vi "Micro-PL v10.1.0.vi"() -> ()   [LabVIEW 2010]
uses:
  drivers/Oxford ITC/ITCAPPS.LLB/ITCSetup.ctl
  drivers/Oxford ITC/ITCSUBS.LLB/ITCIO.ctl
  drivers/Oxford ITC/BUSGEN.LLB/OxfordAddress.ctl
  drivers/Oxford ITC/ITCSUBS.LLB/ITCVersion.ctl
  subvi/ESA-C/TypeDefs/ESA-C Live Controls.ctl
  subvi/ESA-C/TypeDefs/ESA-C Current Values.ctl
  subvi/ESA-C/TypeDefs/ESA-C Connection Settings.ctl
  subvi/ESA-C/TypeDefs/ESA-C Set Positions.ctl
  subvi/ITC503/TypeDefs/ITC503 Settings.ctl
  subvi/ITC503/TypeDefs/ITC503 Current Values.ctl
  subvi/iHR550/TypeDefs/iHR Current Values.ctl
  subvi/iHR550/TypeDefs/iHR Settings.ctl
  subvi/Mapping/TypeDefs/Mapping Spectra Params.ctl
  <vilib>/Utility/miscctls.llb/LVPointTypeDef.ctl
  drivers/Horiba Spectrum One 3000V/Lib/CCD_command.llb/Comm Params.ctl
panel:
  out "Int. Time Temp":dbl
  out "Wavelengths (nm)":dbl[](array[numeric])
  out "Measurement Running":bool
  out "ITC503s Running":bool
  out "Drive Running":bool
  out "CCD3500V Running":bool
  out "iHR550 Running":bool
  in  "Exit":bool
  out "iHR550 Status":bool
  out "Drive Status":bool
  out "CCD3500V Status":bool
  out "ITC503 Status":bool
  in  "CCD3500V Connection":T1={"Comm Interface"=1, "BUS"=0, "Address"=5, "Com Port"=0}
  out "Video Running":bool
  out "iHR550 RefNum":refnum<k7> caption="Mono RefNum out"
  out "ITC Setup":T2={"Description"="", "IO Info"={"Address"={"Com Port"=1, "ISOBUS Address"=1, "GPIB Address"=24, "Communication"=enum."ISOBUS"}, "Version"=enum."ITC503", "Ch 1 dec places"=1, "Ch 2 dec places"=1, "Ch 3 dec places"=1, "Ch1 Name"="", "Ch2 Name"="", "Ch3 Name"=""}}
  in  "Register":T6(tab)
  in  "iHR550 Force Init":bool=TRUE
  in  "iHR550 Connect":bool
  in  "iHR550 ID":string(combo)="iHR550" caption="Monochromator ID"
  out "ITC503 Current Values":T7 {"ITC503 Gradient" format="%.2f"; "ITC503 Setpoint" min=-273.0 max=300000.0 step=0.0001 format="%.1f"; "ITC503 I" format="%_1f"; "ITC503 P" format="%_1f"; "ITC503 Temperature" min=0.0 max=1645.0 step=1e-05 format="%.2f"; "ITC503 Heater" min=0.0 max=100.0 step=0.01 scale=0.0..100.0}
  in  "ITC503 Settings":T8={"ITC503 Set Setpoint"=0.0, "ITC503 Set Auto Heater"=TRUE, "ITC503 Set Auto PID"=TRUE, "P"=0.0, "I"=0.0, "D"=0.0} {"D" min=0.0 max=100.0 step=0.1 format="%.1f"; "I" min=0.0 max=100.0 step=0.1 format="%.1f"; "P" min=0.0 max=100.0 step=0.1 format="%.1f"; "ITC503 Set Setpoint" min=-273.0 max=300000.0 step=0.1 format="%.1f"}
  in  "ITC503 Configure":bool
  in  "ITC503 Connect":bool
  in  "ITC503 Selector":u16(ring) caption="Select Device" items=["ITC503s"]
  out "Drive Current Values":T9 {"Position"."Drive Z Position" min=-273.0 max=300000.0 step=0.0001 format="%.1f"; "Position"."Drive Y Position" min=-273.0 max=300000.0 step=0.0001 format="%.1f"; "Position"."Drive X Position" min=-273.0 max=300000.0 step=0.0001 format="%.1f"; "Voltages"."Drive Z Voltage" min=-273.0 max=300000.0 step=0.0001 format="%.1f"; "Voltages"."Drive Y Voltage" min=-273.0 max=300000.0 step=0.0001 format="%.1f"; "Voltages"."Drive X Voltage" min=-273.0 max=300000.0 step=0.0001 format="%.1f"}
  in  "Drive Connection":T10={"Objective GPIB-Port"=4, "Stage GPIB-Port"=4, "Drive Selector"=0, "Drive Velocity (V/s)"=5.0} {"Drive Velocity (V/s)" min=10.0 max=160.0 step=0.1 format="%.1f"; "Drive Selector" items=["Obj.", "Stage"]; "Stage GPIB-Port" min=1 max=20 step=1 format="%#.0f"; "Objective GPIB-Port" min=1 max=20 step=1 format="%#.0f"}
  in  "Drive Connect":bool
  out "CCD3500 Temperature":dbl caption="Temp. (°C)" min=10.0 max=160.0 step=0.1 format="%.1f"
  in  "CCD3500V GPIB-Port":i32=5 caption="GPIB-Port" min=1 max=20 step=1 format="%#.0f"
  in  "CCD3500V Connect":bool
  in  "CCD3000 Current Rep.":string="0/0"
  in  "Spectrum Load":bool
  in  "Spectrum Save":bool
  out "Spectrum":cluster{dbl[], dbl[]}[](graph)
  in  "Video Show":bool
  in  "Drive GoTo":bool caption="Objective Move Abs."
  in  "Drive New Positions":T11 {"Drive X Set" min=10.0 max=160.0 step=0.1 format="%.1f"; "Drive Z Set" min=10.0 max=160.0 step=0.1 format="%.1f"; "Drive Y Set" min=10.0 max=160.0 step=0.1 format="%.1f"}
  in  "Spectrum Autosave":bool=TRUE caption="iHR550 Force Init"
  in  "CCD3500 Preview":bool
  in  "CCD3500 Acquire":bool
  in  "Spectra Settings":T12={"Integration Time"=1.0, "Repetitions"=1, "Mapping Spectra"=TRUE} caption="Mapping Spectra Settings" {"Repetitions" min=1 max=100 step=1; "Integration Time" min=0.1 max=6000.0 step=0.1 format="%.1f"}
  in  "Mapping Start":bool
  in  "iHR550 Configure":bool
  in  "iHR Settings":T13={"iHR550 Set Exit Mirror"=2, "iHR550 Set Side Exit"=0.0, "iHR550 Set Front Entrance"=0.0, "iHR550 Set Wavelength"=897.9988, "iHR550 Set Grating"=0, "iHR550 Set Grating Switch"=FALSE, "iHR550 Set Wavelength Switch"=FALSE, "iHR550 Set Mirror Switch"=FALSE, "iHR550 Set Slits Switch"=FALSE} {"iHR550 Set Grating" items=["1800"=1, "600"=2, "150"=3]; "iHR550 Set Wavelength" min=0.0 max=1500.0 step=1.0; "iHR550 Set Side Exit" min=0.0 max=2000.0 step=1.0; "iHR550 Set Exit Mirror" items=["Front"=2, "Side"=3]}
  out "iHR Current Values":T14={"iHR 550 Front Entrance"=0.0, "iHR550 Side Exit"=0.0, "iHR550 Wavelength"=897.9988, "iHR550 Exit Mirror"=2, "iHR550 Grating"="1", "Grating Index"=1} {"iHR550 Exit Mirror" items=["EntranceMirror", "ExitMirror", "Front", "Side"]}
  out "Drive Live Current Values":T9 {"Position"."Drive Z Position" min=-273.0 max=300000.0 step=0.0001 format="%.1f"; "Position"."Drive Y Position" min=-273.0 max=300000.0 step=0.0001 format="%.1f"; "Position"."Drive X Position" min=-273.0 max=300000.0 step=0.0001 format="%.1f"; "Voltages"."Drive Z Voltage" min=-273.0 max=300000.0 step=0.0001 format="%.1f"; "Voltages"."Drive Y Voltage" min=-273.0 max=300000.0 step=0.0001 format="%.1f"; "Voltages"."Drive X Voltage" min=-273.0 max=300000.0 step=0.0001 format="%.1f"}
  in  "Drive Live Controls":T15={"Snapshot"=FALSE, "Move Step"=1.0, "Move Home"=FALSE, "Move Down"=FALSE, "Move Up"=FALSE, "Move Left"=FALSE, "Move Right"=FALSE, "Move Out"=FALSE, "Move In"=FALSE} {"Move Step" min=0.0 max=30.0 step=0.1 format="%.1f"}
  # "Correlation Setup"
  # "Active"
  # "Active"
  # "ITC"
  # "iHR"
  # "Drive"
  # "CCD"
  # "Status"
  # "CCD"
  # "ITC"
  # "iHR"
  # "Drive"
  # "Monochromator"
  # "Cryostat"
  # "Drives"
  # "CCD-Camera"
  # "Drive Control"
  # "Spectrum"
  # "CCD"
  # "Mapping"
  # "Launch the Spectral Mapping VI and Raman Tool Set 2.0 in a new window."
  # "Monochromator"
  # "XY"
  # "Z"
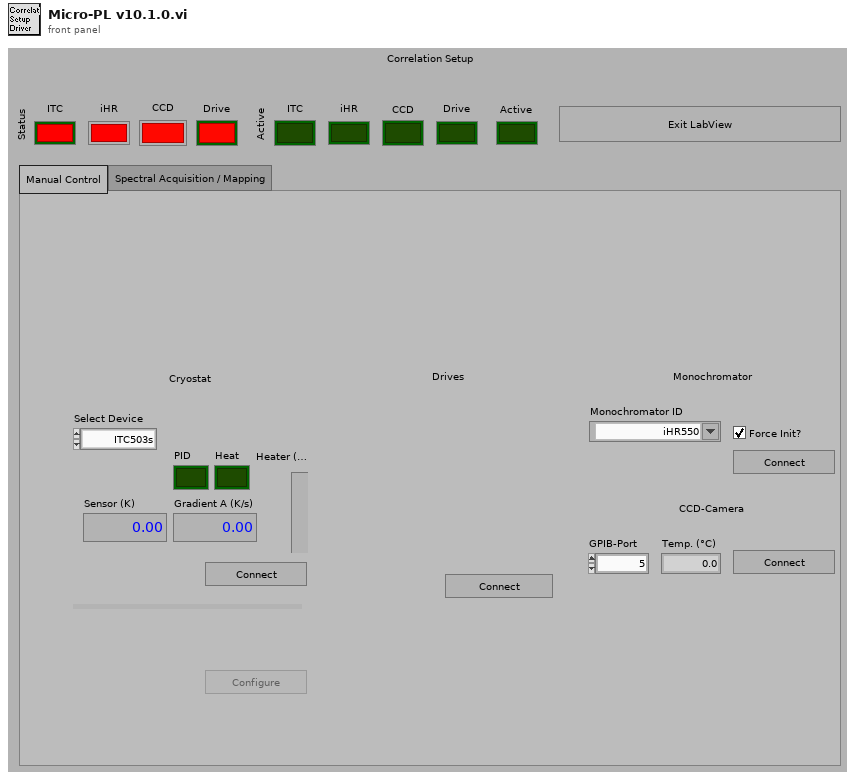
[diagram p1: front panel]
types:
  T1 = cluster{"Comm Interface":u16, "BUS":i16, "Address":i16, "Com Port":i32}
  T2 = typedef "ITCSetup.ctl" = cluster{"Description":string, "IO Info":T3}
  T3 = typedef "ITCIO.ctl" = cluster{"Address":T4, "Version":T5, "Ch 1 dec places":i16, "Ch 2 dec places":i16, "Ch 3 dec places":i16, "Ch1 Name":string, "Ch2 Name":string, "Ch3 Name":string}
  T4 = typedef "OxfordAddress.ctl" = cluster{"Com Port":i32, "ISOBUS Address":i32, "GPIB Address":i16, "Communication":enum16{"RS232", "ISOBUS", "GPIB", "Gateway"}}
  T5 = typedef "ITCVersion.ctl" = enum16{"ITC502", "ITC503", "ITC601"}
  T6 = enum32{"Manual Control", "Spectral Acquisition / Mapping"}
  T7 = typedef "ITC503 Current Values.ctl" = cluster{"ITC503 Heater":dbl, "ITC503 Temperature":dbl, "ITC503 P":dbl, "ITC503 I":dbl, "ITC503 D":dbl, "ITC503 Setpoint":dbl, "ITC503 Gradient":dbl, "ITC503 Heater Auto":bool, "ITC503 PID Auto":bool}
  T8 = typedef "ITC503 Settings.ctl" = cluster{"ITC503 Set Setpoint":dbl, "ITC503 Set Auto Heater":bool, "ITC503 Set Auto PID":bool, "P":dbl, "I":dbl, "D":dbl}
  T9 = typedef "ESA-C Current Values.ctl" = cluster{"Voltages":cluster{"Drive X Voltage":dbl, "Drive Y Voltage":dbl, "Drive Z Voltage":dbl}, "Position":cluster{"Drive X Position":dbl, "Drive Y Position":dbl, "Drive Z Position":dbl}}
  T10 = typedef "ESA-C Connection Settings.ctl" = cluster{"Objective GPIB-Port":i32, "Stage GPIB-Port":i32, "Drive Selector":u16, "Drive Velocity (V/s)":dbl}
  T11 = typedef "ESA-C Set Positions.ctl" = cluster{"Drive X Set":dbl, "Drive Y Set":dbl, "Drive Z Set":dbl}
  T12 = typedef "Mapping Spectra Params.ctl" = cluster{"Integration Time":dbl, "Repetitions":u16, "Mapping Spectra":bool}
  T13 = typedef "iHR Settings.ctl" = cluster{"iHR550 Set Exit Mirror":u16, "iHR550 Set Side Exit":dbl, "iHR550 Set Front Entrance":dbl, "iHR550 Set Wavelength":dbl, "iHR550 Set Grating":u16, "iHR550 Set Grating Switch":bool, "iHR550 Set Wavelength Switch":bool, "iHR550 Set Mirror Switch":bool, "iHR550 Set Slits Switch":bool}
  T14 = typedef "iHR Current Values.ctl" = cluster{"iHR 550 Front Entrance":dbl, "iHR550 Side Exit":dbl, "iHR550 Wavelength":dbl, "iHR550 Exit Mirror":i32, "iHR550 Grating":string, "Grating Index":i32}
  T15 = typedef "ESA-C Live Controls.ctl" = cluster{"Snapshot":bool, "Move Step":dbl, "Move Home":bool, "Move Down":bool, "Move Up":bool, "Move Left":bool, "Move Right":bool, "Move Out":bool, "Move In":bool}
  T16 = typedef "LVPointTypeDef.ctl" = cluster{"Horizontal":i16, "Vertical":i16}
  T17 = enum16{"CCD Temperature Z345", "CCD Temperature Z308", "CCD Gain"}
  T18 = enum8{"Enabled", "Disabled", "Disabled and Grayed Out"}
  T19 = typedef "Comm Params.ctl" = cluster{"Comm Interface":u16, "BUS":i16, "Address":i16, "Com Port":i32}
  T20 = cluster{"CCD3000 Connection":T19, "Drive Connection Settings":T10, "ITC503 Current Values":T7, "Wavelengths (nm)":dbl[], "Drive Current Values":T9, "iHR Current Values":T14, "Spectra Settings":T12, "CCD3500 Temperature":dbl, "Simulate Drive 2":bool, "Simulate Spectra 2":bool}
  T21 = cluster{"Intensities":dbl[], "Wavelengths":dbl[]}[]
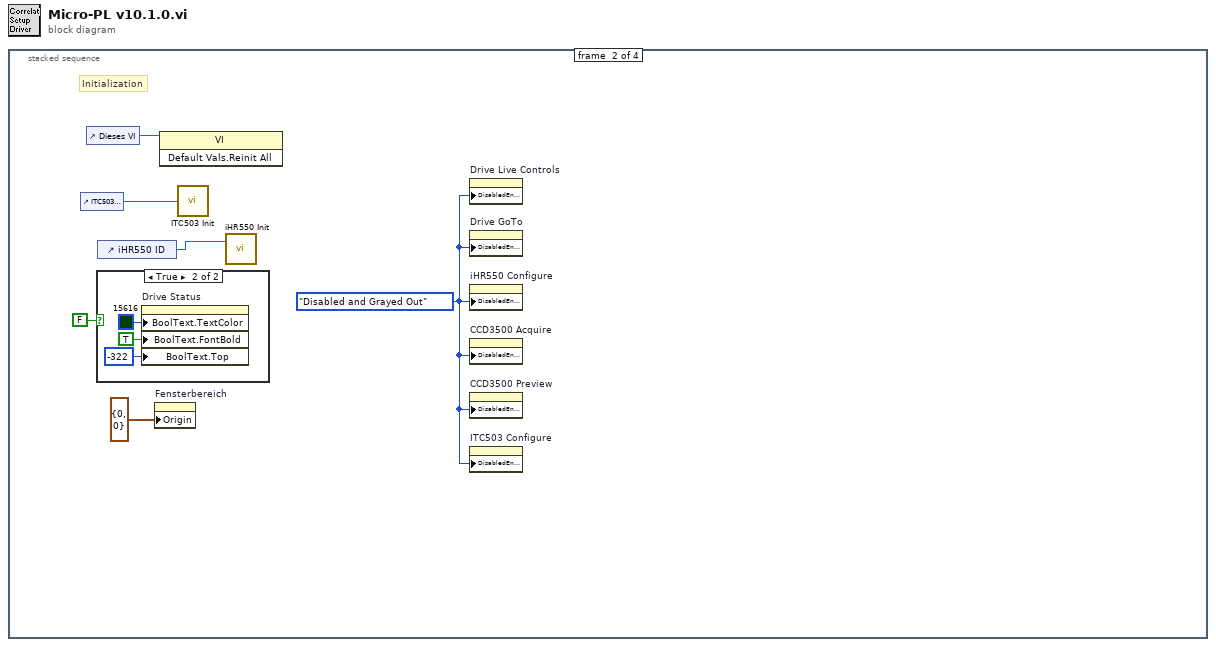
[diagram p0: block diagram]
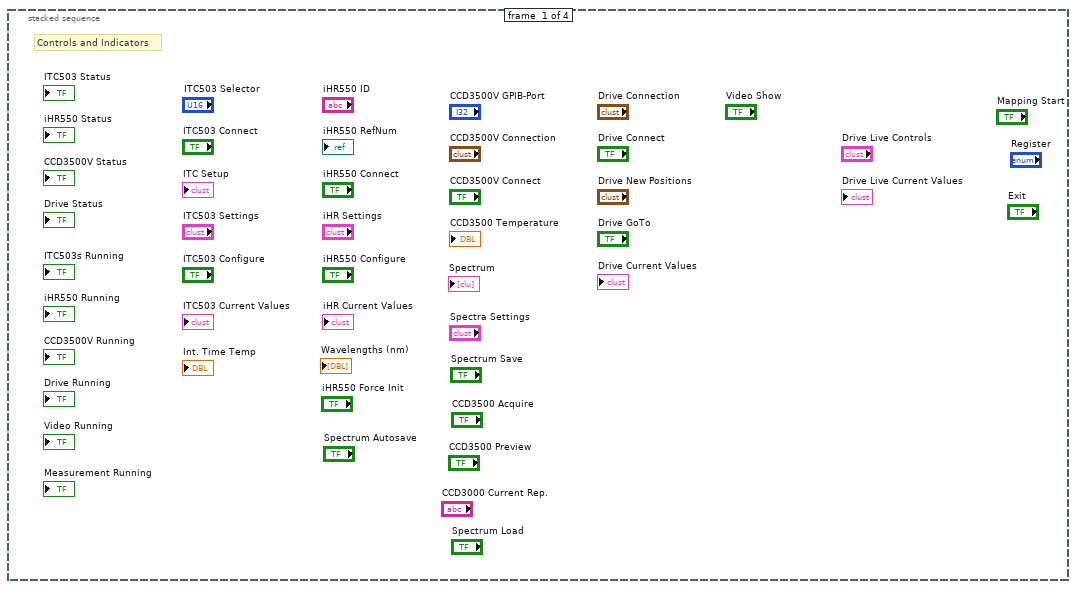
[diagram p2: hidden frame]
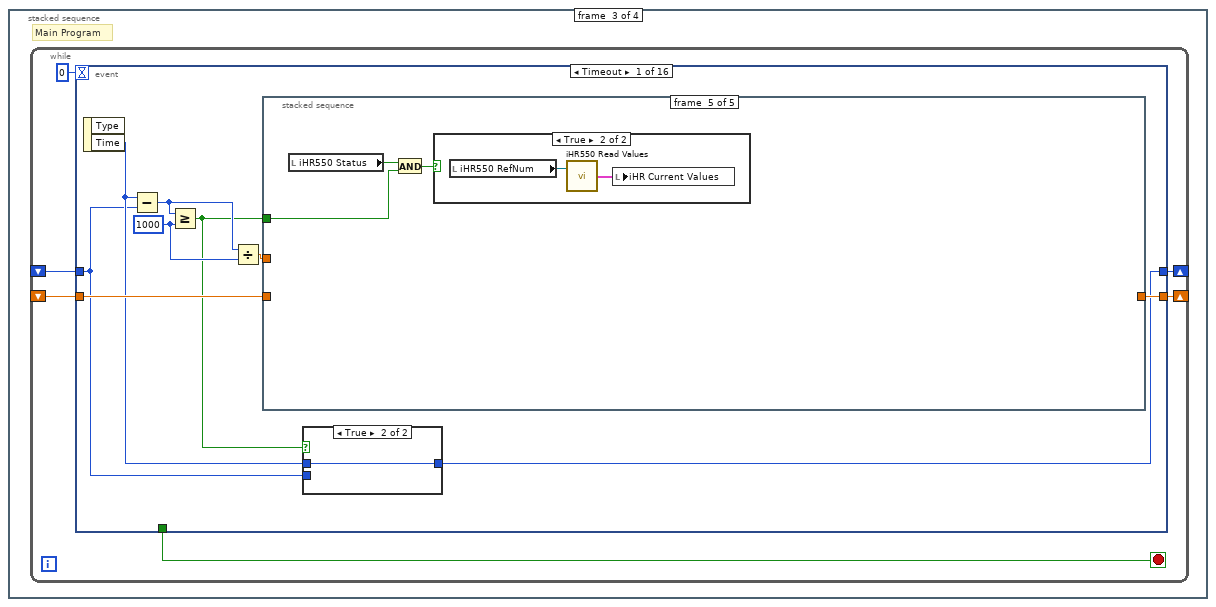
[diagram p4: hidden frame]
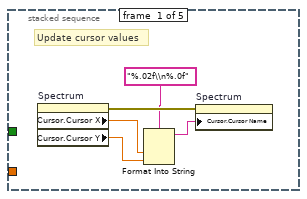
[diagram p6: hidden frame]
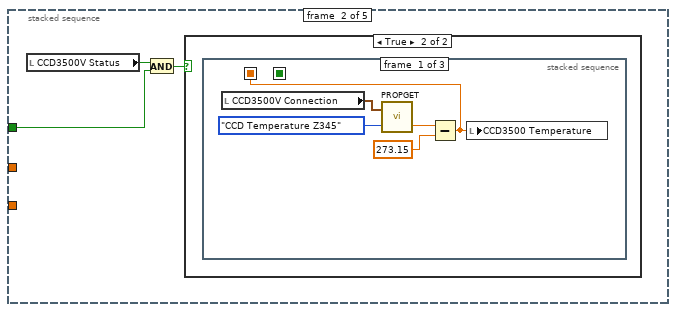
[diagram p7: hidden frame]
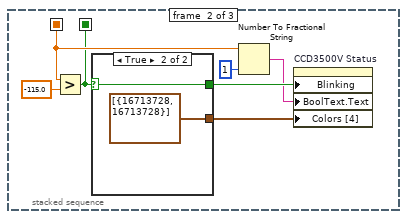
[diagram p9: hidden frame]
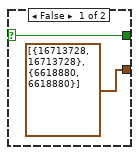
[diagram p10: hidden frame]
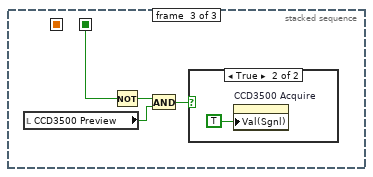
[diagram p11: hidden frame]
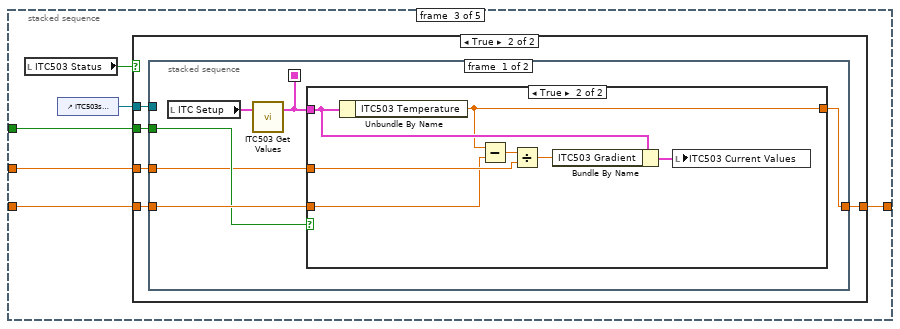
[diagram p13: hidden frame]
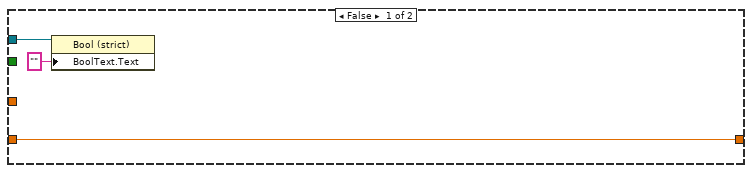
[diagram p14: hidden frame]
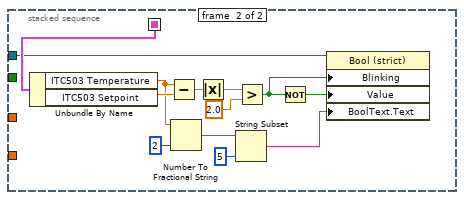
[diagram p16: hidden frame]
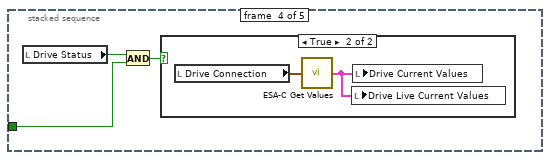
[diagram p17: hidden frame]
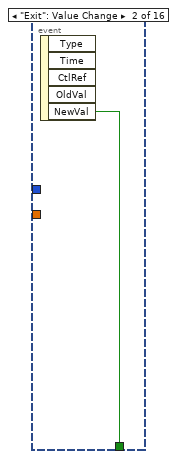
[diagram p20: hidden frame]
diagram:
  n1 = stacked-sequence {
    frame #0 {
      # "Controls and Indicators"
    }
    frame #1 {
      w1 = T18."Disabled and Grayed Out" ("Deaktiviert")
      # "Initialization"
      n2 = control-ref of="ITC503 Selector"() -> (w6:refnum<vi>)
      n3 = control-ref of="Dieses VI"() -> (w5:refnum<vi>)
      n4 = case shown="True" FALSE {
        frame False {
        }
        frame True {
          n5 = property on="Drive Status" class="Bool (strict)"("BoolText.TextColor"=u32 15616, "BoolText.FontBold"=TRUE ("Boolescher Text.Schriftart:Fett"), "BoolText.Top"=-322 ("Boolescher Text.Position:Oben")) -> ()  [unwired: 2 in, 2 out]
        }
      }
      n6 = control-ref of="iHR550 ID"() -> (w4:refnum<vi>)
      n7 = property on="Fensterbereich" class="Pane"("Origin"=T16 {"Horizontal"=0, "Vertical"=0}) -> ()  [unwired: 2 in, 2 out]
      n8 = invoke class="VI" method="Default Vals.Reinit All"(reference=w5) -> ()  [unwired: 2 in, 3 out]
      n9 = call "ITC503 Init.vi"("ITC Selector"=w6) -> ()  [unwired: 1 in]
      n10 = call "iHR550 Init.vi"("Mono ID"=w4) -> ()  [unwired: 2 in]
      n11 = property on="Drive Live Controls" class="Clust (strict)"("DisabledEnum"=w1) -> ()  [unwired: 2 in, 2 out]
      n12 = property on="Drive GoTo" class="Bool (strict)"("DisabledEnum"=w1) -> ()  [unwired: 2 in, 2 out]
      n13 = property on="iHR550 Configure" class="Bool (strict)"("DisabledEnum"=w1) -> ()  [unwired: 2 in, 2 out]
      n14 = property on="CCD3500 Acquire" class="Bool (strict)"("DisabledEnum"=w1) -> ()  [unwired: 2 in, 2 out]
      n15 = property on="CCD3500 Preview" class="Bool (strict)"("DisabledEnum"=w1) -> ()  [unwired: 2 in, 2 out]
      n16 = property on="ITC503 Configure" class="Bool (strict)"("DisabledEnum"=w1) -> ()  [unwired: 2 in, 2 out]
    }
    frame #2 {
      # "Main Program"
      n17 = while "Main-Program" {
        shift-right: [w13] -> _
        shift-left: _ -> [w12]
        shift-right: [w11] -> _
        shift-left: _ -> [w10]
        stop <- w15 stop-if-true
        n18 = event shown="[0] Timeout" {
          selector: _ -> [_ _ _ _ _ _ _ _ _ _ _ _ _ _ _ _]
          dyn-events: _ -> [_ _ _ _ _ _ _ _ _ _ _ _ _ _ _ _]
          timeout: 0 -> [_ _ _ _ _ _ _ _ _ _ _ _ _ _ _ _]
          tunnel: [_ w107 _ _ _ _ _ _ _ _ _ _ _ _ _ _] -> w15
          tunnel: w12 -> [w16 _ _ _ _ _ _ _ _ _ _ _ _ _ _ _]
          tunnel: [w17 _ _ _ _ _ _ _ _ _ _ _ _ _ _ _] -> w13
          tunnel: [w24 _ _ _ _ _ _ _ _ _ _ _ _ _ _ _] -> w11
          tunnel: w10 -> [w23 _ _ _ _ _ _ _ _ _ _ _ _ _ _ _]
          event Timeout {
            w21 = u32 1000 ("y")
            n19 = event-data() -> ("Time"=w18:u32)  [unwired: 1 in, 1 out]
            n20 = Subtract(x=w18, y=w16) -> (x-y=w22:u32)
            n21 = Greater Or Equal?(x=w22, y=w21) -> (x >= y?=w19:bool)
            n22 = Divide(x=w22, y=w21) -> (x/y=w20:dbl)
            n23 = stacked-sequence {
              tunnel: [_ _ w59 _ _] -> w24
              tunnel: w23 -> [_ _ w58 _ _]
              tunnel: w19 -> [_ w32 w57 w99 w103]
              tunnel: w20 -> [_ _ w56 _ _]
              frame #0 {
                # "Update cursor values"
                n24 = property on="Spectrum" class="XYGraph (strict)"() -> (error out=w31:errorcluster, "Cursor.Cursor X"=w30:dbl, "Cursor.Cursor Y"=w29:dbl)  [unwired: 2 in, 1 out]
                n25 = Format Into String(format string="%.02f\\n%.0f", w30, w29) -> (resulting string=w27:string)  [unwired: 2 in, 1 out]
                n26 = property on="Spectrum" class="XYGraph (strict)"(error in=w31, "Cursor.Cursor Name"=w27) -> ()  [unwired: 1 in, 2 out]
              }
              frame #1 {
                n27 = local read "CCD3500V Status"() -> (w34:bool)
                n28 = And(x=w34, y=w32) -> (x .and. y?=w33:bool)
                n29 = case shown="True" w33 {
                  frame False {
                  }
                  frame True {
                    n30 = stacked-sequence {
                      seq-local: [w35 _ _] -> [_ w44 _]
                      seq-local: [_ w40 _] -> [_ _ w54]
                      frame #0 {
                        n31 = local read "CCD3500V Connection"() -> (w39:T1)
                        n32 = call "PROPGET.VI"("CCD Prop ID"=T17."CCD Temperature Z345", "Comm Params"=w39) -> ("Output Param"=w37:dbl)  [unwired: 1 out]
                        n33 = Subtract(x=w37, y=273.15) -> (x-y=w35:dbl)
                        n34 = local write "CCD3500 Temperature"(w35) -> ()
                      }
                      frame #1 {
                        n35 = Greater?(x=w44, y=-115.0) -> (0:w40:bool)
                        n36 = case shown="True" w40 {
                          selector: w40 -> [w48 w50]
                          tunnel: [cluster{u32, u32}[] [{16713728, 16713728}, {6618880, 6618880}] ("Farben [4]") cluster{u32, u32}[] [{16713728, 16713728}] ("Farben [4]")] -> w41
                          tunnel: [w48 w50] -> w43
                          frame False {
                          }
                          frame True {
                          }
                        }
                        n37 = Number To Fractional String(number=w44, precision (6)=i16 1 ("Genauigkeit (6)")) -> (F-format string=w42:string)  [unwired: 2 in]
                        n38 = property on="CCD3500V Status" class="Bool (strict)"("Blinking"=w43, "BoolText.Text"=w42, "Colors [4]"=w41) -> ()  [unwired: 2 in, 2 out]
                      }
                      frame #2 {
                        n39 = local read "CCD3500 Preview"() -> (w52:bool)
                        n40 = Not(x=w54) -> (.not. x?=w53:bool)
                        n41 = And(x=w53, y=w52) -> (x .and. y?=w51:bool)
                        n42 = case shown="True" w51 {
                          frame False {
                          }
                          frame True {
                            n43 = property on="CCD3500 Acquire" class="Bool (strict)"("Val(Sgnl)"=TRUE ("Wert (signalisierend)")) -> ()  [unwired: 2 in, 2 out]
                          }
                        }
                      }
                    }
                  }
                }
              }
              frame #2 {
                n44 = local read "ITC503 Status"() -> (w61:bool)
                n45 = control-ref of="ITC503s Running"() -> (w60:refnum<vi>)
                n46 = case shown="True" w61 {
                  tunnel: w60 -> [w64 w69]
                  tunnel: [w62 w68] -> w59
                  tunnel: w58 -> [w62 w67]
                  tunnel: w57 -> [_ w66]
                  tunnel: w56 -> [_ w65]
                  frame False {
                    n47 = property class="Bool (strict)"(reference=w64, "BoolText.Text"="" ("Boolescher Text.Text")) -> ()  [unwired: 1 in, 2 out]
                  }
                  frame True {
                    n48 = stacked-sequence {
                      seq-local: [w74 _] -> [_ w92]
                      tunnel: w69 -> [_ w89]
                      tunnel: [w73 _] -> w68
                      tunnel: w67 -> [w72 _]
                      tunnel: w66 -> [w71 _]
                      tunnel: w65 -> [w70 _]
                      frame #0 {
                        n49 = local read "ITC Setup"() -> (w75:T2)
                        n50 = call "ITC503 Get Values.vi"("ITC Setup"=w75) -> ("ITC503 Current Values"=w74:T7)  [unwired: 1 in, 1 out]
                        n51 = case shown="True" w71 {
                          tunnel: w74 -> [_ w80]
                          tunnel: [w76 w79] -> w73
                          tunnel: w72 -> [w76 w77]
                          tunnel: w70 -> [_ w78]
                          frame False {
                          }
                          frame True {
                            n52 = Unbundle By Name(w80) -> ("ITC503 Temperature"=w79:dbl)
                            n53 = Subtract(x=w79, y=w77) -> (x-y=w82:dbl)
                            n54 = Divide(x=w82, y=w78) -> (x/y=w83:dbl)
                            n55 = Bundle By Name(cluster=w80, "ITC503 Gradient"=w83) -> (w81:T7)
                            n56 = local write "ITC503 Current Values"(w81) -> ()
                          }
                        }
                      }
                      frame #1 {
                        n57 = Unbundle By Name(w92) -> ("ITC503 Temperature"=w88:dbl, "ITC503 Setpoint"=w93:dbl)
                        n58 = Subtract(x=w88, y=w93) -> (x-y=w94:dbl)
                        n59 = Number To Fractional String(number=w88, precision (6)=i16 2 ("Genauigkeit (6)")) -> (F-format string=w86:string)  [unwired: 2 in]
                        n60 = Absolute Value(x=w94) -> (abs(x)=w95:dbl)
                        n61 = String Subset(string=w86, length (rest)=5 ("Länge (Rest)")) -> (substring=w84:string)  [unwired: 1 in]
                        n62 = Greater?(x=w95, y=2.0) -> (0:w91:bool)
                        n63 = Not(x=w91) -> (.not. x?=w90:bool)
                        n64 = property class="Bool (strict)"(reference=w89, "Blinking"=w91, "Value"=w90, "BoolText.Text"=w84) -> ()  [unwired: 1 in, 2 out]
                      }
                    }
                  }
                }
              }
              frame #3 {
                n65 = local read "Drive Status"() -> (w98:bool)
                n66 = And(x=w98, y=w99) -> (x .and. y?=w97:bool)
                n67 = case shown="True" w97 {
                  frame False {
                  }
                  frame True {
                    n68 = local read "Drive Connection"() -> (w100:T10)
                    n69 = call "ESA-C Get Values.vi"("Drive Connection Settings"=w100) -> ("Drive Current Values"=w101:T9)
                    n70 = local write "Drive Live Current Values"(w101) -> ()
                    n71 = local write "Drive Current Values"(w101) -> ()
                  }
                }
              }
              frame #4 {
                n72 = local read "iHR550 Status"() -> (w104:bool)
                n73 = And(x=w104, y=w103) -> (x .and. y?=w102:bool)
                n74 = case shown="True" w102 {
                  frame False {
                  }
                  frame True {
                    n75 = local read "iHR550 RefNum"() -> (w106:refnum<k7>)
                    n76 = call "iHR550 Read Values.vi"("JYMONOLib.IJYMonoReqd"=w106) -> ("iHR Current Values"=w105:T14)  [unwired: 1 in]
                    n77 = local write "iHR Current Values"(w105) -> ()
                  }
                }
              }
            }
            n78 = case shown="True" w19 {
              tunnel: w18 -> [_ w26]
              tunnel: [w25 w26] -> w17
              tunnel: w16 -> [w25 _]
              frame False {
              }
              frame True {
              }
            }
          }
          event "Exit": Value Change {
            n79 = event-data() -> ("NewVal"=w107:bool)  [unwired: 1 in, 4 out]
          }
          event "ITC503 Connect": Value Change {
            n80 = event-data() -> ("NewVal"=w108:bool)  [unwired: 1 in, 4 out]
            n81 = stacked-sequence {
              tunnel: w108 -> [_ w110 _]
              frame #0 {
                n82 = property on="ITC503s Running" class="Bool (strict)"("Blinking"=TRUE ("Blinkend")) -> ()  [unwired: 2 in, 2 out]
              }
              frame #1 {
                n83 = case shown="True" w110 {
                  selector: w110 -> [w115 _]
                  tunnel: [w115 w122] -> w112
                  frame False {
                    # "disconnect"
                    n84 = control-ref of="ITC503s Running"() -> (w116:refnum<vi>)
                    n85 = property class="Bool (strict)"(reference=w116, "Blinking"=w115, "Value"=w115) -> ()  [unwired: 1 in, 2 out]
                  }
                  frame True {
                    # "connect"
                    n86 = local read "ITC503 Selector"() -> (w123:u16)
                    n87 = call "ITC503 Connect.vi"("ITC Selector"=w123) -> ("ITC Setup"=w121:T2, "Connected"=w122:bool)
                    n88 = local write "ITC Setup"(w121) -> ()
                    n89 = call "ITC503 Get Values.vi"("ITC Setup"=w121) -> ("ITC503 Current Values"=w120:T7)  [unwired: 1 in, 1 out]
                    n90 = Unbundle By Name(w120) -> ("ITC503 Setpoint"=w117:dbl)
                    n91 = Bundle By Name(cluster=T8 {"ITC503 Set Setpoint"=0.0, "ITC503 Set Auto Heater"=TRUE, "ITC503 Set Auto PID"=TRUE, "P"=0.0, "I"=0.0, "D"=0.0} ("ITC503 Settings"), "ITC503 Set Setpoint"=w117) -> (w118:T8)
                    n92 = local write "ITC503 Settings"(w118) -> ()
                  }
                }
                n93 = case shown="False" w112 {
                  tunnel: [T18."Disabled and Grayed Out" ("Deaktiviert") T18."Enabled" ("Deaktiviert")] -> w111
                  frame False {
                  }
                  frame True {
                  }
                }
                n94 = local write "ITC503 Status"(w112) -> ()
                n95 = local write "ITC503 Connect"(w112) -> ()
                n96 = property on="ITC503 Configure" class="Bool (strict)"("DisabledEnum"=w111) -> ()  [unwired: 2 in, 2 out]
              }
              frame #2 {
                n97 = property on="ITC503s Running" class="Bool (strict)"("Blinking"=FALSE ("Blinkend")) -> ()  [unwired: 2 in, 2 out]
              }
            }
          }
          event "iHR550 Connect": Value Change {
            n98 = event-data() -> ("NewVal"=w125:bool)  [unwired: 1 in, 4 out]
            n99 = stacked-sequence {
              tunnel: w125 -> [_ w128 _]
              frame #0 {
                n100 = property on="iHR550 Running" class="Bool (strict)"("Blinking"=TRUE ("Blinkend")) -> ()  [unwired: 2 in, 2 out]
              }
              frame #1 {
                n101 = case shown="True" w128 {
                  selector: w128 -> [w132 _]
                  tunnel: [w132 w145] -> w127
                  frame False {
                    # "disconnect"
                  }
                  frame True {
                    # "connect"
                    n102 = local read "iHR550 Force Init"() -> (w143:bool)
                    n103 = control-ref of="iHR550 Set Grating"() -> (w144:refnum<vi>)
                    n104 = local read "iHR550 ID"() -> (w146:string)
                    n105 = call "iHR550 Connect.vi"("Force\nInitialization"=w143, "Grating Selector"=w144, "Mono ID"=w146) -> ("Initialized"=w145:bool, "iHR550 RefNum"=w142:refnum<k7>)  [unwired: 2 in, 4 out]
                    n106 = local write "iHR550 RefNum"(w142) -> ()
                    n107 = call "iHR550 Read Values.vi"("JYMONOLib.IJYMonoReqd"=w142) -> ("iHR Current Values"=w134:T14)  [unwired: 1 in]
                    n108 = local write "iHR Current Values"(w134) -> ()
                    n109 = Unbundle By Name(w134) -> ("iHR 550 Front Entrance"=w140:dbl, "iHR550 Side Exit"=w139:dbl, "iHR550 Wavelength"=w138:dbl, "iHR550 Exit Mirror"=w137:i32, "Grating Index"=w135:i32)
                    n110 = call "iHR550 Convert Axis.vi"("iHR Current Values"=w134) -> ("Wavelengths (nm)"=w133:dbl[])
                    n111 = local write "Wavelengths (nm)"(w133) -> ()
                    n112 = Bundle By Name(cluster=T13 {"iHR550 Set Exit Mirror"=0, "iHR550 Set Side Exit"=0.0, "iHR550 Set Front Entrance"=0.0, "iHR550 Set Wavelength"=0.0, "iHR550 Set Grating"=0, "iHR550 Set Grating Switch"=FALSE, "iHR550 Set Wavelength Switch"=FALSE, "iHR550 Set Mirror Switch"=FALSE, "iHR550 Set Slits Switch"=FALSE} ("iHR Settings"), "iHR550 Set Front Entrance"=w140, "iHR550 Set Side Exit"=w139, "iHR550 Set Wavelength"=w138, "iHR550 Set Exit Mirror"=w137, "iHR550 Set Grating"=w135) -> (w136:T13)
                    n113 = local write "iHR Settings"(w136) -> ()
                  }
                }
                n114 = local write "iHR550 Status"(w127) -> ()
                n115 = local write "iHR550 Connect"(w127) -> ()
                n116 = case shown="False" w127 {
                  tunnel: [T18."Disabled and Grayed Out" ("Deaktiviert") T18."Enabled" ("Deaktiviert")] -> w129
                  frame False {
                  }
                  frame True {
                  }
                }
                n117 = property on="iHR550 Configure" class="Bool (strict)"("DisabledEnum"=w129) -> ()  [unwired: 2 in, 2 out]
              }
              frame #2 {
                n118 = property on="iHR550 Running" class="Bool (strict)"("Blinking"=FALSE ("Blinkend")) -> ()  [unwired: 2 in, 2 out]
                n119 = local write "iHR550 Force Init"(FALSE ("iHR550 Force Init")) -> ()
              }
            }
          }
          event "CCD3500V Connect": Value Change {
            n120 = event-data() -> ("NewVal"=w149:bool)  [unwired: 1 in, 4 out]
            n121 = stacked-sequence {
              tunnel: w149 -> [_ w151 _]
              frame #0 {
                n122 = property on="CCD3500V Running" class="Bool (strict)"("Blinking"=TRUE ("Blinkend")) -> ()  [unwired: 2 in, 2 out]
              }
              frame #1 {
                n123 = case shown="True" w151 {
                  selector: w151 -> [w157 _]
                  tunnel: [w157 w158] -> w153
                  frame False {
                    # "disconnect"
                    n124 = local read "CCD3500V Connection"() -> (w156:T1)
                    n125 = call "CCDSTOP.VI"("Comm Params"=w156) -> ()  [unwired: 1 out]
                  }
                  frame True {
                    # "connect"
                    n126 = stacked-sequence {
                      seq-local: [_ w162 _] -> [_ _ w164]
                      tunnel: [_ w163 _] -> w158
                      frame #0 {
                        n127 = local read "CCD3500V GPIB-Port"() -> (w160:i32)
                        n128 = Bundle By Name(cluster=T19 {"Comm Interface"=1, "BUS"=0, "Address"=5, "Com Port"=1} ("Comm Params"), "Address"=w160) -> (w161:T19)
                        n129 = local write "CCD3500V Connection"(w161) -> ()
                      }
                      frame #1 {
                        n130 = local read "CCD3500V Connection"() -> (w162:T1)
                        n131 = call "CCD3000 Initialize.vi"("Comm Params"=w162) -> ("Success"=w163:bool)  [unwired: 9 in, 1 out]
                      }
                      frame #2 {
                        n132 = local read "Spectra Settings"() -> (w165:T12)
                        n133 = Unbundle By Name(w165) -> ("Integration Time"=w166:dbl)
                        n134 = local write "Int. Time Temp"(w166) -> ()
                        n135 = call "CCD3000 Prepare Acquisition.vi"("Mapping Spectra Settings"=w165, "Comm Params"=w164) -> ()  [unwired: 4 in]
                      }
                    }
                  }
                }
                n136 = local write "CCD3500V Connect"(w153) -> ()
                n137 = local write "CCD3500V Status"(w153) -> ()
                n138 = case shown="False" w153 {
                  tunnel: [T18."Disabled and Grayed Out" ("Deaktiviert") T18."Enabled" ("Deaktiviert")] -> w152
                  frame False {
                  }
                  frame True {
                  }
                }
                n139 = property on="CCD3500V Status" class="Bool (strict)"("BoolText.Visible"=w153) -> ()  [unwired: 2 in, 2 out]
                n140 = property on="CCD3500 Acquire" class="Bool (strict)"("DisabledEnum"=w152) -> ()  [unwired: 2 in, 2 out]
                n141 = property on="CCD3500 Preview" class="Bool (strict)"("DisabledEnum"=w152) -> ()  [unwired: 2 in, 2 out]
              }
              frame #2 {
                n142 = property on="CCD3500V Running" class="Bool (strict)"("Blinking"=FALSE ("Blinkend")) -> ()  [unwired: 2 in, 2 out]
              }
            }
          }
          event "Drive Connect": Value Change {
            n143 = event-data() -> ("NewVal"=w168:bool)  [unwired: 1 in, 4 out]
            n144 = stacked-sequence {
              tunnel: w168 -> [_ w172 _]
              frame #0 {
                n145 = property on="Drive Running" class="Bool (strict)"("Blinking"=TRUE ("Blinkend")) -> ()  [unwired: 2 in, 2 out]
              }
              frame #1 {
                n146 = local read "Drive Connection"() -> (w173:T10)
                n147 = Not(x=w172) -> (.not. x?=w174:bool)
                n148 = call "ESA-C Connect.vi"("Remote=F /Local=T"=w174, "Drive Connection Settings"=w173) -> ("Success"=w175:bool)  [unwired: 2 in]
                n149 = Exclusive Or(1:w174, 2:w175) -> (0:w176:bool)
                n150 = local write "Drive Connect"(w176) -> ()
                n151 = local write "Drive Status"(w176) -> ()
                n152 = case shown="False" w176 {
                  tunnel: [T18."Disabled and Grayed Out" ("Deaktiviert") T18."Enabled" ("Deaktiviert")] -> w171
                  tunnel: ["" ("Boolescher Text.Text") w179] -> w170
                  frame False {
                  }
                  frame True {
                    n153 = property on="Drive Selector" class="Ring (strict)"() -> ("RingText.Text"=w179:string)  [unwired: 2 in, 2 out]
                  }
                }
                n154 = property on="Drive Live Controls" class="Clust (strict)"("DisabledEnum"=w171) -> ()  [unwired: 2 in, 2 out]
                n155 = property on="Drive Status" class="Bool (strict)"("BoolText.Text"=w170) -> ()  [unwired: 2 in, 2 out]
                n156 = property on="Drive GoTo" class="Bool (strict)"("DisabledEnum"=w171) -> ()  [unwired: 2 in, 2 out]
              }
              frame #2 {
                n157 = property on="Drive Running" class="Bool (strict)"("Blinking"=FALSE ("Blinkend")) -> ()  [unwired: 2 in, 2 out]
              }
            }
          }
          event "Video Show": Value Change {
            n158 = event-data() -> ("NewVal"=w182:bool)  [unwired: 1 in, 4 out]
            n159 = case shown="False" w182 {
              frame False {
                n160 = call "Video Close.vi"() -> ()  [unwired: 11 in, 1 out]
              }
              frame True {
                n161 = call "Video Open.vi"() -> ()  [unwired: 11 in, 1 out]
              }
            }
          }
          event "ITC503 Configure": Value Change {
            n162 = event-data() -> ("NewVal"=w183:bool)  [unwired: 1 in, 4 out]
            n163 = stacked-sequence {
              tunnel: w183 -> [_ w185 _]
              frame #0 {
                n164 = property on="ITC503s Running" class="Bool (strict)"("Blinking"=TRUE ("Blinkend")) -> ()  [unwired: 2 in, 2 out]
              }
              frame #1 {
                n165 = local read "ITC503 Status"() -> (w187:bool)
                n166 = And(x=w187, y=w185) -> (x .and. y?=w186:bool)
                n167 = case shown="True" w186 {
                  frame False {
                  }
                  frame True {
                    n168 = local read "ITC503 Settings"() -> (w188:T8)
                    n169 = local read "ITC Setup"() -> (w189:T2)
                    n170 = call "ITC503 Set Values.vi"("Set Channel"=i16 1, "ITC503 Settings"=w188, "ITC Setup"=w189) -> ()  [unwired: 2 in]
                  }
                }
              }
              frame #2 {
                w191 = FALSE ("Blinkend")
                n171 = local write "ITC503 Configure"(w191) -> ()
                n172 = property on="ITC503s Running" class="Bool (strict)"("Blinking"=w191) -> ()  [unwired: 2 in, 2 out]
              }
            }
          }
          event "iHR550 Configure": Value Change {
            n173 = event-data() -> ("NewVal"=w192:bool)  [unwired: 1 in, 4 out]
            n174 = stacked-sequence {
              tunnel: w192 -> [_ w194 _]
              frame #0 {
                n175 = property on="iHR550 Running" class="Bool (strict)"("Blinking"=TRUE ("Blinkend")) -> ()  [unwired: 2 in, 2 out]
              }
              frame #1 {
                n176 = local read "iHR550 Status"() -> (w196:bool)
                n177 = local read "iHR550 RefNum"() -> (w197:refnum<k7>)
                n178 = And(x=w196, y=w194) -> (x .and. y?=w195:bool)
                n179 = case shown="True" w195 {
                  tunnel: w197 -> [_ w198]
                  frame False {
                  }
                  frame True {
                    n180 = stacked-sequence {
                      seq-local: [_ w203 _] -> [_ _ w206]
                      tunnel: w198 -> [w199 w204 _]
                      frame #0 {
                        w202 = u16 2 items=["Front"=2, "Side"=3] ("Entrance Mirror")
                        n181 = local read "iHR Settings"() -> (w200:T13)
                        n182 = call "iHR550 Set Values.vi"("Refnum out"=w199, "Entrance Mirror"=w202, "Target\nSide Entrance"=0.0 ("Target\nSide Entrance"), "iHR Settings"=w200) -> ()  [unwired: 11 in, 1 out]
                      }
                      frame #1 {
                        n183 = call "iHR550 Read Values.vi"("JYMONOLib.IJYMonoReqd"=w204) -> ("iHR Current Values"=w203:T14)  [unwired: 1 in]
                        n184 = local write "iHR Current Values"(w203) -> ()
                      }
                      frame #2 {
                        n185 = call "iHR550 Convert Axis.vi"("iHR Current Values"=w206) -> ("Wavelengths (nm)"=w205:dbl[])
                        n186 = local write "Wavelengths (nm)"(w205) -> ()
                      }
                    }
                  }
                }
              }
              frame #2 {
                w207 = FALSE ("Blinkend")
                n187 = local write "iHR550 Configure"(w207) -> ()
                n188 = property on="iHR550 Running" class="Bool (strict)"("Blinking"=w207) -> ()  [unwired: 2 in, 2 out]
              }
            }
          }
          event "CCD3500 Preview": Value Change {
            n189 = event-data() -> ("NewVal"=w208:bool)  [unwired: 1 in, 4 out]
            n190 = case shown="True" w208 {
              frame False {
              }
              frame True {
                n191 = property on="CCD3500 Acquire" class="Bool (strict)"("Val(Sgnl)"=TRUE ("Wert (signalisierend)")) -> ()  [unwired: 2 in, 2 out]
              }
            }
          }
          event "CCD3500 Acquire": Value Change {
            n192 = event-data() -> ("NewVal"=w210:bool)  [unwired: 1 in, 4 out]
            n193 = stacked-sequence {
              tunnel: w210 -> [w211 _]
              frame #0 {
                n194 = case shown="True" w211 {
                  frame False {
                  }
                  frame True {
                    n195 = local read "CCD3500V Connection"() -> (w212:T1)
                    n196 = local read "Spectra Settings"() -> (w213:T12)
                    n197 = stacked-sequence {
                      tunnel: w213 -> [w216 w228 _]
                      tunnel: w212 -> [w215 w224 _]
                      frame #0 {
                        # "prepare acquisition if settings changed"
                        n198 = Unbundle By Name(w216) -> ("Integration Time"=w214:dbl)
                        n199 = local read "Int. Time Temp"() -> (w217:dbl)
                        n200 = Equal?(x=w214, y=w217) -> (x = y?=w218:bool)
                        n201 = case shown="False" w218 {
                          tunnel: w217 -> [_ _]
                          tunnel: w216 -> [w221 _]
                          tunnel: w215 -> [w220 _]
                          tunnel: w214 -> [w219 _]
                          frame False {
                            n202 = local write "Int. Time Temp"(w219) -> ()
                            n203 = call "CCD3000 Prepare Acquisition.vi"("Mapping Spectra Settings"=w221, "Comm Params"=w220) -> ()  [unwired: 4 in]
                          }
                          frame True {
                          }
                        }
                      }
                      frame #1 {
                        n204 = local read "CCD3500 Preview"() -> (w227:bool)
                        n205 = Unbundle By Name(w228) -> ("Repetitions"=w225:u16)
                        n206 = Select(t=i8 1, s=w227, f=w225) -> (s? t:f=w223:u16)
                        n207 = for {
                          N: w223 -> [w233]
                          tunnel: w224 -> [w245]
                          shift-right: [w240] -> _
                          shift-left: u16[][] [] -> [w243]
                          i -> [w234]
                          stop <- w239 continue-if-true
                          n208 = control-ref of="CCD3500 Acquire"() -> (w238:refnum<vi>)
                          n209 = control-ref of="CCD3500V Running"() -> (w237:refnum<vi>)
                          n210 = call "CCD3000 Spectral Acquisition.vi"("Acquire"=w238, "Running"=w237, "Comm Params"=w245) -> ("Raw-Spectrum"=w244:u16[])  [unwired: 6 in, 2 out]
                          n211 = Number To Decimal String(number=w233) -> (decimal integer string=w232:string)  [unwired: 1 in]
                          n212 = Build Array (concatenate)(w244, w243) -> (w240:u16[][])
                          n213 = Increment(x=w234) -> (x+1=w230:i32)
                          n214 = Number To Decimal String(number=w230) -> (decimal integer string=w231:string)  [unwired: 1 in]
                          n215 = local read "Wavelengths (nm)"() -> (w242:dbl[])
                          n216 = Concatenate Strings(w231, "/" ("string"), w232) -> (w236:string)
                          n217 = call "CCD3000 Average Spectra.vi"("Repetitions"=w230, "Raw Spectra"=w240) -> ("Raw Spectrum"=w241:dbl[])
                          n218 = local read "CCD3500 Acquire"() -> (w239:bool)
                          n219 = local write "CCD3000 Current Rep."(w236) -> ()
                          n220 = call "CCD3000 Pixel to Wavelength v10.1.0.vi"("Wavelengths (nm)"=w242, "Raw Spectrum"=w241) -> ("Spectrum-Cluster"=w229:T21)  [unwired: 1 out]
                          n221 = local write "Spectrum"(w229) -> ()
                        }
                      }
                      frame #2 {
                        n222 = local read "Spectrum Autosave"() -> (w246:bool)
                        n223 = case shown="True" w246 {
                          frame False {
                          }
                          frame True {
                            n224 = property on="Spectrum Save" class="Bool (strict)"("Val(Sgnl)"=TRUE ("Value (Signaling)")) -> ()  [unwired: 2 in, 2 out]
                          }
                        }
                      }
                    }
                  }
                }
              }
              frame #1 {
                n225 = local write "CCD3500 Acquire"(FALSE ("Blinkend")) -> ()
                n226 = local write "CCD3000 Current Rep."("0/0" ("CCD3000 Current Rep.")) -> ()
              }
            }
          }
          event "Drive GoTo": Value Change {
            n227 = event-data() -> ("NewVal"=w250:bool)  [unwired: 1 in, 4 out]
            n228 = stacked-sequence {
              tunnel: w250 -> [_ w252 _]
              frame #0 {
                n229 = property on="Drive Running" class="Bool (strict)"("Blinking"=TRUE ("Blinkend")) -> ()  [unwired: 2 in, 2 out]
              }
              frame #1 {
                n230 = local read "Drive Status"() -> (w254:bool)
                n231 = And(x=w254, y=w252) -> (x .and. y?=w253:bool)
                n232 = case shown="True" w253 {
                  frame False {
                  }
                  frame True {
                    n233 = local read "Drive New Positions"() -> (w255:T11)
                    n234 = local read "Drive Connection"() -> (w256:T10)
                    n235 = control-ref of="Drive Running"() -> (w257:refnum<vi>)
                    n236 = call "ESA-C Move Absolute.vi"("Running"=w257, "Drive New Abs. Positions"=w255, "Drive Connection Settings"=w256) -> ()  [unwired: 2 in]
                  }
                }
              }
              frame #2 {
                w258 = FALSE ("Blinkend")
                n237 = local write "Drive GoTo"(w258) -> ()
                n238 = property on="Drive Running" class="Bool (strict)"("Blinking"=w258) -> ()  [unwired: 2 in, 2 out]
              }
            }
          }
          event Value Change {
            n239 = event-data() -> ("NewVal"=w260:bool)  [unwired: 1 in, 4 out]
            n240 = local read "Drive Status"() -> (w261:bool)
            n241 = And(x=w261, y=w260) -> (x .and. y?=w259:bool)
            n242 = case shown="True" w259 {
              frame False {
              }
              frame True {
                n243 = stacked-sequence {
                  seq-local: [w262 _] -> [_ w283]
                  frame #0 {
                    # "Move and Read"
                    n244 = flat-sequence {
                      tunnel: [w271] -> w267
                      tunnel: [w269] -> w266
                      tunnel: [w268] -> w265
                      tunnel: w267 -> [w273]
                      tunnel: w266 -> [w275]
                      tunnel: [w275] -> w264
                      tunnel: w265 -> [w274]
                      tunnel: [w272] -> w263
                      tunnel: w264 -> [w282]
                      tunnel: w263 -> [w280]
                      tunnel: [w280] -> w262
                      frame #0 {
                        n245 = local read "Drive Live Controls"() -> (w268:T15)
                        n246 = local read "Drive Connection"() -> (w269:T10)
                        n247 = control-ref of="Drive Running"() -> (w270:refnum<vi>)
                        n248 = call "ESA-C Live Control.vi"("Running"=w270, "Drive Live Controls"=w268, "Drive Connection Settings"=w269) -> ("Reset Switches"=w271:bool)  [unwired: 1 in]
                      }
                      frame #1 {
                        n249 = case shown="True" w273 {
                          tunnel: w274 -> [w276 w279]
                          tunnel: [w276 w278] -> w272
                          frame False {
                          }
                          frame True {
                            w277 = FALSE ("Move Out")
                            n250 = Bundle By Name(cluster=w279, "Move Home"=w277, "Move Down"=w277, "Move Up"=w277, "Move Left"=w277, "Move Right"=w277, "Move Out"=w277, "Move In"=w277) -> (w278:T15)
                          }
                        }
                      }
                      frame #2 {
                        n251 = local write "Drive Live Controls"(w280) -> ()
                        n252 = call "ESA-C Get Values.vi"("Drive Connection Settings"=w282) -> ("Drive Current Values"=w281:T9)
                        n253 = local write "Drive Live Current Values"(w281) -> ()
                      }
                    }
                  }
                  frame #1 {
                    # "Snapshot"
                    n254 = Unbundle By Name(w283) -> ("Snapshot"=w286:bool)
                    n255 = case shown="True" w286 {
                      selector: w286 -> [w287 _]
                      tunnel: [w287 FALSE] -> w285
                      frame False {
                      }
                      frame True {
                        n256 = call "Video Snapshot.vi"() -> ()  [unwired: 11 in, 1 out]
                      }
                    }
                    n257 = Bundle By Name(cluster=w283, "Snapshot"=w285) -> (w284:T15)
                    n258 = local write "Drive Live Controls"(w284) -> ()
                  }
                }
              }
            }
          }
          event "Spectrum Save": Value Change {
            n259 = event-data() -> ("NewVal"=w289:bool)  [unwired: 1 in, 4 out]
            n260 = stacked-sequence {
              tunnel: w289 -> [w290 _]
              frame #0 {
                n261 = case shown="True" w290 {
                  frame False {
                  }
                  frame True {
                    n262 = local read "Spectrum"() -> (w293:cluster{dbl[], dbl[]}[])
                    n263 = local read "CCD3500 Temperature"() -> (w297:dbl)
                    n264 = local read "ITC503 Current Values"() -> (w298:T7)
                    n265 = local read "Drive Current Values"() -> (w299:T9)
                    n266 = local read "iHR Current Values"() -> (w301:T14)
                    n267 = local read "Spectra Settings"() -> (w300:T12)
                    n268 = Index Array(array=w293, index=0 ("Index")) -> (element=w291:cluster{dbl[], dbl[]})
                    n269 = Unbundle(w291) -> (w304:dbl[], w303:dbl[])
                    n270 = Build Array(w304, w303) -> (w302:dbl[][])
                    n271 = call "Export_spectrumFileName.vi"("ITC503 Current Values"=w298, "iHR Current Values"=w301, "Spectra Settings"=w300, "Drive Current Values"=w299, "CCD3500 Temperature"=w297) -> ("Filename"=w296:string)
                    n272 = local read "Spectrum Autosave"() -> (w294:bool)
                    n273 = call "Export_2DtoTxt.vi"("Auto?"=w294, "Data (2D)"=w302, "Export Type"="Spectrum", "Filename"=w296) -> ()  [unwired: 2 in]
                  }
                }
              }
              frame #1 {
                n274 = local write "Spectrum Save"(FALSE ("Spectrum Save")) -> ()
              }
            }
          }
          event "Spectrum Load": Value Change {
            n275 = event-data() -> ("NewVal"=w306:bool)  [unwired: 1 in, 4 out]
            n276 = stacked-sequence {
              tunnel: w306 -> [w307 _]
              frame #0 {
                n277 = case shown="True" w307 {
                  frame False {
                  }
                  frame True {
                    n278 = local read "Spectrum"() -> (w310:cluster{dbl[], dbl[]}[])
                    n279 = call "Load Spectrum.vi"() -> ("Graph Cluster"=w308:cluster{dbl[], dbl[]})  [unwired: 3 in, 2 out]
                    n280 = Build Array (concatenate)(w310, w308) -> (w309:cluster{dbl[], dbl[]}[])
                    n281 = local write "Spectrum"(w309) -> ()
                  }
                }
              }
              frame #1 {
                n282 = local write "Spectrum Load"(FALSE ("Spectrum Load")) -> ()
              }
            }
          }
          event "Mapping Start": Value Change {
            n283 = event-data() -> ("NewVal"=w312:bool)  [unwired: 1 in, 4 out]
            n284 = case shown="True" w312 {
              frame False {
              }
              frame True {
                n285 = stacked-sequence {
                  frame #0 {
                    n286 = property on="Measurement Running" class="Bool (strict)"("Blinking"=TRUE ("Blinkend")) -> ()  [unwired: 2 in, 2 out]
                  }
                  frame #1 {
                    w328 = FALSE ("Simulate Drive")
                    n287 = local read "CCD3500V Connection"() -> (w324:T1)
                    n288 = local read "CCD3500 Temperature"() -> (w326:dbl)
                    n289 = local read "ITC503 Current Values"() -> (w321:T7)
                    n290 = local read "Drive Current Values"() -> (w319:T9)
                    n291 = local read "iHR Current Values"() -> (w320:T14)
                    n292 = local read "Wavelengths (nm)"() -> (w322:dbl[])
                    n293 = local read "Drive Connection"() -> (w323:T10)
                    n294 = local read "CCD3500V Status"() -> (w315:bool)
                    n295 = local read "Spectra Settings"() -> (w325:T12)
                    n296 = local read "Drive Status"() -> (w317:bool)
                    n297 = Not(x=w317) -> (.not. x?=w316:bool)
                    n298 = Not(x=w315) -> (.not. x?=w314:bool)
                    n299 = Bundle By Name(cluster=T20 {"CCD3000 Connection"={"Comm Interface"=1, "BUS"=0, "Address"=5, "Com Port"=1}, "Drive Connection Settings"={"Objective GPIB-Port"=4, "Stage GPIB-Port"=4, "Drive Selector"=0, "Drive Velocity (V/s)"=5.0}, "ITC503 Current Values"={"ITC503 Heater"=0.0, "ITC503 Temperature"=0.0, "ITC503 P"=0.0, "ITC503 I"=0.0, "ITC503 D"=0.0, "ITC503 Setpoint"=0.0, "ITC503 Gradient"=0.0, "ITC503 Heater Auto"=FALSE, "ITC503 PID Auto"=FALSE}, "Wavelengths (nm)"=[], "Drive Current Values"={"Voltages"={"Drive X Voltage"=0.0, "Drive Y Voltage"=0.0, "Drive Z Voltage"=0.0}, "Position"={"Drive X Position"=0.0, "Drive Y Position"=0.0, "Drive Z Position"=0.0}}, "iHR Current Values"={"iHR 550 Front Entrance"=0.0, "iHR550 Side Exit"=0.0, "iHR550 Wavelength"=897.9988, "iHR550 Exit Mirror"=2, "iHR550 Grating"="1", "Grating Index"=1}, "Spectra Settings"={"Integration Time"=1.0, "Repetitions"=1, "Mapping Spectra"=TRUE}, "CCD3500 Temperature"=0.0, "Simulate Drive 2"=FALSE, "Simulate Spectra 2"=FALSE} ("Input Parameters"), "CCD3000 Connection"=w324, "Drive Connection Settings"=w323, "ITC503 Current Values"=w321, "Wavelengths (nm)"=w322, "Drive Current Values"=w319, "iHR Current Values"=w320, "Spectra Settings"=w325, "CCD3500 Temperature"=w326, "Simulate Drive 2"=w316, "Simulate Spectra 2"=w314) -> (w327:T20)
                    n300 = call "Mapping v10.1.0.vi"("Simulate Spectra"=w328, "Simulate Drive"=w328, "Input Parameters"=w327) -> ()  [unwired: 9 in]
                  }
                  frame #2 {
                    w329 = FALSE ("Mapping Start")
                    n301 = local write "Mapping Start"(w329) -> ()
                    n302 = property on="Measurement Running" class="Bool (strict)"("Blinking"=w329) -> ()  [unwired: 2 in, 2 out]
                  }
                }
              }
            }
          }
        }
      }
    }
    frame #3 {
      # "Close Connections"
      n303 = control-ref of="Dieses VI"() -> (w330:refnum<vi>)
      n304 = invoke class="VI" method="Default Vals.Reinit All"(reference=w330) -> ()  [unwired: 2 in, 3 out]
    }
  }
